vi "Update Add Step Associations Table for Spartan 5.2.vi"(8 "error in (no error)":errorcluster, 11 "Connection Refnum":T1) -> (0 "error out":errorcluster, 3 "Connection Refnum":T1)   [LabVIEW 2011]
uses:
  Summitek EXT/ODBC/SQL Controls/Connection Refnum.ctl
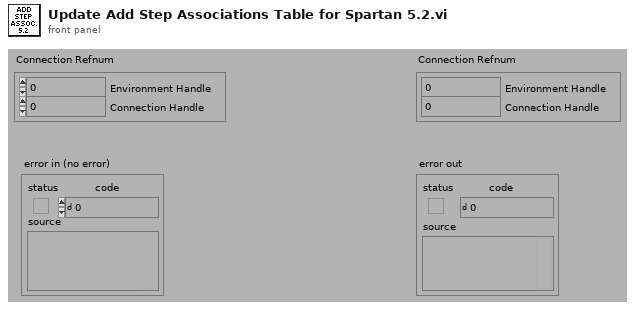
[diagram p1: front panel]
types:
  T1 = typedef "Connection Refnum.ctl" = cluster{"Environment Handle":i32, "Connection Handle":i32}
  T2 = typedef "Statement Refnum.ctl" = cluster{"Statement Handle":i32, "Parameter Number":u16}
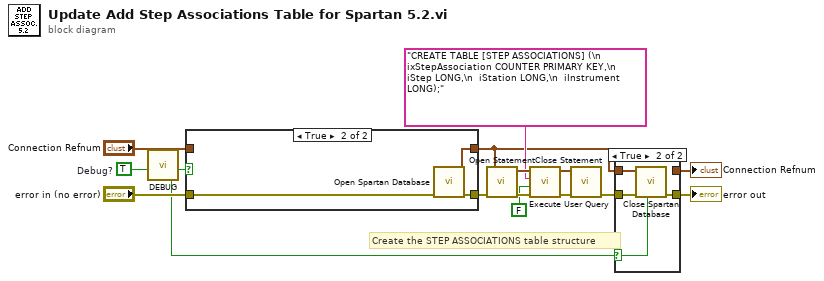
[diagram p0: block diagram]
diagram:
  w12 = TRUE  # Debug?
  # "Create the STEP ASSOCIATIONS table structure"
  n1 = call "DEBUG.vi"("Dev DEBUG? (f)"=w12) -> ("DEBUG?"=w10:bool)  [unwired: 1 in, 5 out]
  n2 = case shown="True" w10 {
    tunnel: "Connection Refnum" -> [w17 _]
    tunnel: "error in (no error)" -> [w16 w20]
    tunnel: [w16 w19] -> w7
    tunnel: [w17 w18] -> w4
    frame False {
    }
    frame True {
      n3 = call "Open Spartan Database.vi"("error in (no error)"=w20) -> ("error out"=w19:errorcluster, "Connection Refnum"=w18:T1)  [unwired: 2 in, 7 out]
    }
  }
  n4 = call "Open Statement.vi"("error in (no error)"=w7, "Connection Refnum"=w4) -> ("error out"=w9:errorcluster, "Statement Refnum"=w8:T2)  [unwired: 4 out]
  n5 = call "Execute User Query.vi"("error in (no error)"=w9, "Return Data? (f)"=FALSE, "User Query"="CREATE TABLE [STEP ASSOCIATIONS] (\n  ixStepAssociation COUNTER PRIMARY KEY,\n  iStep LONG,\n  iStation LONG,\n  iInstrument LONG);", "Statement Refnum"=w8) -> ("error out"=w1:errorcluster, "Statement Refnum"=w2:T2)  [unwired: 2 out]
  n6 = call "Close Statement.vi"("error in (no error)"=w1, "Statement Refnum"=w2) -> ("error out"=w3:errorcluster)  [unwired: 5 out]
  n7 = case shown="True" w10 {
    selector: w10 -> [_ w23]
    tunnel: w3 -> [w22 w26]
    tunnel: [w21 _] -> w11
    tunnel: [w22 w25] -> w13
    tunnel: w4 -> [w21 w24]
    frame False {
    }
    frame True {
      n8 = call "Close Spartan Database.vi"("Force Close? (f)"=w23, "error in (no error)"=w26, "Connection Refnum"=w24) -> ("error out"=w25:errorcluster)  [unwired: 2 in, 6 out]
    }
  }
  "Connection Refnum" <- w11
  "error out" <- w13
